vi "detSetpointFromProfile.vi"(8 "error in (no error)":errorcluster, 11 "Model in":refnum<class "Model.lvclass">) -> (0 "error out":errorcluster, 2 "temperatureSetpoint":dbl[unit]=273.15, 3 "Model out":refnum<class "Model.lvclass">)   [LabVIEW 2013, in "Model.lvclass"]
uses:
  Model.lvclass
  Model.lvclass/Model.ctl
  ApplicationElements/TestMonitor/TestMonitor.lvclass
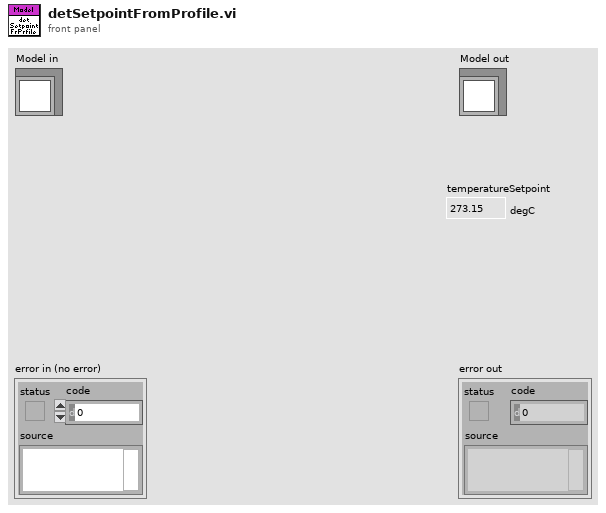
[diagram p1: front panel]
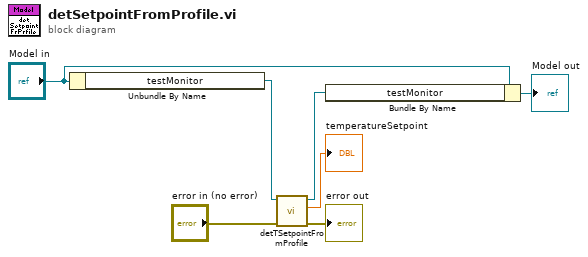
[diagram p0: block diagram]
diagram:
  n1 = Unbundle By Name("Model in") -> ("testMonitor"=w7:refnum<class "TestMonitor.lvclass">)
  n2 = call "detTSetpointFromProfile.vi"("error in (no error)"="error in (no error)", "TestMonitor in"=w7) -> ("error out"=→"error out":errorcluster, "temperatureSetpoint"=→"temperatureSetpoint":dbl[unit], "TestMonitor out"=w6:refnum<class "TestMonitor.lvclass">)  [unwired: 7 in]
  n3 = Bundle By Name(cluster="Model in", "testMonitor"=w6) -> (→"Model out":refnum<class "Model.lvclass">)
